vi "Search Sysdef for Custom Devices.vi"(8 "error in (no error)":errorcluster, 11 "Target Node":refnum<k24>) -> (0 "error out":errorcluster, 1 "Custom Device Names":string[](array[string]), 2 "Custom Device Nodes":refnum<k24>[](array[refnum]), 3 "Target Node Out":refnum<k24>)   [LabVIEW 2011]
uses:
  NationalInstruments.VeriStand.SystemStorage
  <vilib>/ECUMC/NIVS/Support Files.llb/XCPCCP Global.vi
  <vilib>/ECUMC/NIVS/Support Files.llb/XCP and CCP Master Custom Device.lvlib
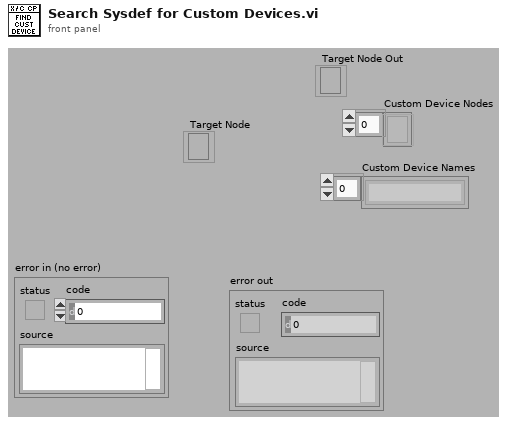
[diagram p1: front panel]
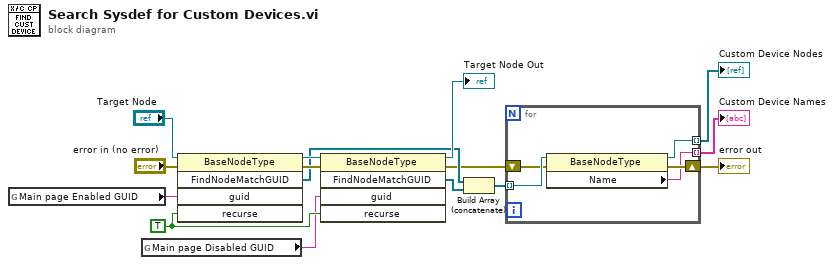
[diagram p0: block diagram]
diagram:
  w14 = TRUE ("recurse")
  n1 = global read "XCPCCP Global.vi" "Main page Enabled GUID"() -> (w11:string)
  n2 = global read "XCPCCP Global.vi" "Main page Disabled GUID"() -> (w13:string)
  n3 = invoke class="BaseNodeType" method="FindNodeMatchGUID"(reference="Target Node", error in="error in (no error)", "guid"=w11, "recurse"=w14) -> (reference out=w15:refnum<k24>, error out=w12:errorcluster, "FindNodeMatchGUID"=w7:refnum<k24>[])  [unwired: 1 in, 2 out]
  n4 = invoke class="BaseNodeType" method="FindNodeMatchGUID"(reference=w15, error in=w12, "guid"=w13, "recurse"=w14) -> (reference out=→"Target Node Out":refnum<k24>, error out=w5:errorcluster, "FindNodeMatchGUID"=w6:refnum<k24>[])  [unwired: 1 in, 2 out]
  n5 = Build Array (concatenate)(w7, w6) -> (w4:refnum<k24>[])
  n6 = for {
    tunnel: w4 -> [w20] mode=indexing
    shift-right: [w18] -> w1
    shift-left: w5 -> [w19]
    tunnel: [w17] -> w3 mode=indexing
    tunnel: [w16] -> w2 mode=indexing
    n7 = property class="BaseNodeType"(reference=w20, error in=w19) -> (reference out=w17:refnum<k24>, error out=w18:errorcluster, "Name"=w16:string)
  }
  "error out" <- w1
  "Custom Device Nodes" <- w3
  "Custom Device Names" <- w2
